vi "Disp.vi"(7 "Event":refnum<user-event>, 8 "error in (no error)":errorcluster, 9 "Digital Input Signals":digitalwaveform[](array[waveform]), 10 "Relay":string, 11 "TCP 380 in":refnum<class "TCP 380.lvclass">) -> (0 "error out":errorcluster)   [LabVIEW 2021, in "TCP 380.lvclass"]
uses:
  TCP 380.lvclass
  TCP 380.lvclass/TCP 380.ctl
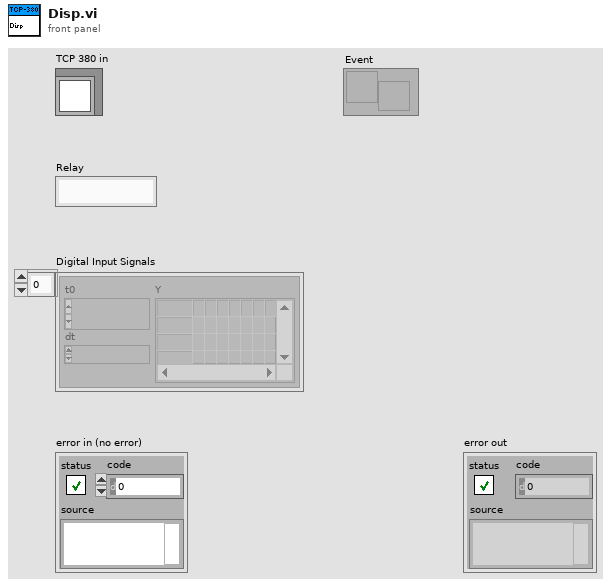
[diagram p1: front panel]
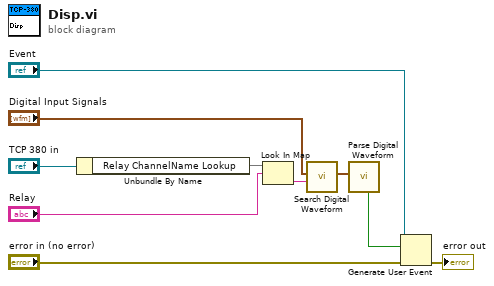
[diagram p0: block diagram]
diagram:
  n1 = Unbundle By Name("TCP 380 in") -> ("Relay ChannelName Lookup"=w6:map{string, string})
  n2 = Look In Map(map=w6, key="Relay") -> (value=w7:string)  [unwired: 1 in, 1 out]
  n3 = call <vilib>:"Search Digital Waveform.vi"("NI_ChannelName"=w7, "Waveforms"="Digital Input Signals") -> ("Waveform"=w10:digitalwaveform)  [unwired: 8 in, 1 out]
  n4 = call <vilib>:"Parse Digital Waveform.vi"("Digital Wave"=w10) -> ("Boolean"=w9:bool)  [unwired: 6 in, 4 out]
  n5 = Generate User Event(user event="Event", event data cluster=w9, error in="error in (no error)") -> (error out=→"error out":errorcluster)  [unwired: 1 in, 1 out]
